vi "Reset DDS.vi"(8 "error in (no error)":errorcluster, 11 "NMR in":refnum<class "NMR.lvclass">) -> (0 "error out":errorcluster, 1 "String as ASCII":string, 3 "NMR out":refnum<class "NMR.lvclass">)   [LabVIEW 2011, in "NMR.lvclass"]
uses:
  NMR.lvclass
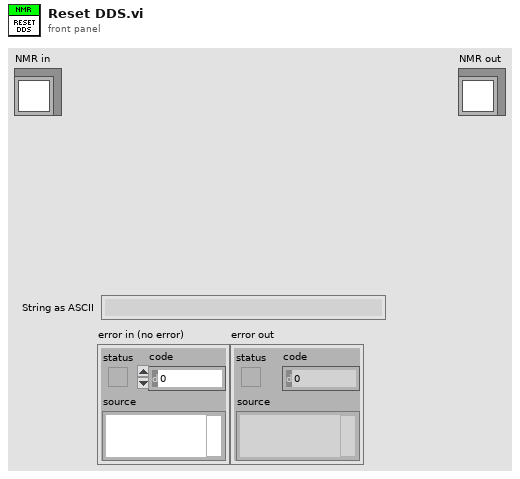
[diagram p1: front panel]
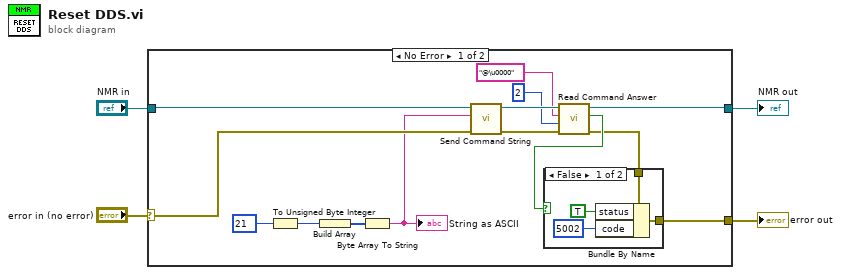
[diagram p0: block diagram]
diagram:
  n1 = case shown="No Error" "error in (no error)" {
    selector: "error in (no error)" -> [w15 w25]
    tunnel: [w7 w25] -> w3
    tunnel: [w16 w24] -> w1
    tunnel: "NMR in" -> [w18 w24]
    frame No Error {
      n2 = To Unsigned Byte Integer(number=u8 21) -> (unsigned 8bit integer=w5:u8)
      n3 = Build Array(w5) -> (w13:u8[])
      n4 = Byte Array To String(unsigned byte array=w13) -> (string=w12:string)
      "String as ASCII" <- w12
      n5 = call-dynamic "Send Command String.vi"("error in (no error)"=w15, "Command String"=w12, "NMR in"=w18) -> ("error out"=w14:errorcluster, "NMR out"=w17:refnum<class "NMR.lvclass">)  [unwired: 7 in]
      n6 = call-dynamic "Read Command Answer.vi"("error in (no error)"=w14, "bytes to read"=u32 2 ("Number bytes Read"), "String Seached"="@\u0000" ("search char"), "NMR in"=w17) -> ("error out"=w8:errorcluster, "Expected Answer?"=w9:bool, "NMR out"=w16:refnum<class "NMR.lvclass">)  [unwired: 5 in]
      n7 = case shown="False" w9 {
        tunnel: w8 -> [w20 w23]
        tunnel: [w19 w23] -> w7
        frame False {
          n8 = Bundle By Name(cluster=w20, "status"=TRUE, "code"=5002) -> (w19:errorcluster)
        }
        frame True {
        }
      }
    }
    frame Error {
    }
  }
  "error out" <- w3
  "NMR out" <- w1
